vi "Version_2.0_Single_Column_Code.vi"() -> ()   [LabVIEW 2020] (continued)
                                n6800 = local read "VISA Refnum in\nfor Pump"() -> (w7287:refnum<visa-resource-name>)
                                n6801 = local write "Valve V5 Open"(FALSE ("Valve V1 Open")) -> ()
                                n6802 = local write "Suction pressure \nfor grid deposition"(w7284) -> ()
                                n6803 = local write "Re-deposit Sample\nonto Grid"(FALSE ("Redeposit Sample\nonto Grid")) -> ()
                                n6804 = local write "Pause Data Collection"(TRUE ("Pause Data Collection")) -> ()
                                n6805 = call "HardStopCurrentProcess (SubVI).vi"("VISA Refnum in"=w7287) -> ()  [unwired: 11 in]
                                n6806 = local write "Valve V6 Open"(TRUE ("Valve V2 Open")) -> ()
                                n6807 = local write "Valve V7 Open"(TRUE ("Valve V3 Open")) -> ()
                                }
                                frame #1 {
                                n6808 = call <vilib>:"fgt init.vi"() -> ("error out"=w7288:errorcluster)  [unwired: 11 in]
                                n6809 = while {
                                tunnel: [w7291] -> w7289
                                tunnel: w7288 -> [w7290]
                                stop <- w7294 stop-if-true
                                # "'5' corresponds to 2nd positin in the line-up series"
                                n6810 = local read "Stop for End of \nExperiment \nand Data Writing"() -> (w7295:bool)
                                n6811 = local read "Suction Pressure\nfor EM-grid \nDeposition (mbar)"() -> (w7292:sgl)
                                n6812 = call <vilib>:"fgt set pressure.vi"("error in (no error)"=w7290, "pressure"=w7292, "pressureIndex"=u32 1) -> ("error out"=w7291:errorcluster)  [unwired: 8 in]
                                n6813 = local read "Suction On/Off"() -> (w7297:bool)
                                n6814 = Not(x=w7297) -> (.not. x?=w7296:bool)
                                n6815 = Wait (ms)(milliseconds to wait=u32 10) -> ()  [unwired: 1 out]
                                n6816 = Or(x=w7296, y=w7295) -> (x .or. y?=w7294:bool)
                                }
                                n6817 = call <vilib>:"fgt close.vi"("error in (no error)"=w7289) -> ()  [unwired: 10 in, 1 out]
                                }
                                frame #2 {
                                n6818 = call <vilib>:"fgt init.vi"() -> ("error out"=w7300:errorcluster)  [unwired: 11 in]
                                n6819 = while {
                                tunnel: w7300 -> [w7303]
                                tunnel: [w7301] -> w7299
                                stop <- w7309 stop-if-true
                                n6820 = local read "Stop for End of \nExperiment \nand Data Writing"() -> (w7305:bool)
                                n6821 = local read "Suction On/Off"() -> (w7307:bool)
                                n6822 = call <vilib>:"fgt set pressure.vi"("error in (no error)"=w7303, "pressure"=sgl 0.0, "pressureIndex"=u32 1) -> ("error out"=w7301:errorcluster)  [unwired: 8 in]
                                n6823 = Not(x=w7307) -> (.not. x?=w7306:bool)
                                n6824 = Wait (ms)(milliseconds to wait=u32 10) -> ()  [unwired: 1 out]
                                n6825 = Or(x=w7306, y=w7305) -> (x .or. y?=w7309:bool)
                                }
                                n6826 = call <vilib>:"fgt close.vi"("error in (no error)"=w7299) -> ()  [unwired: 10 in, 1 out]
                                }
                                frame #3 {
                                n6827 = local write "Valve V7 Open"(FALSE ("Valve V3 Open")) -> ()
                                n6828 = local write "Valve V5 Open"(FALSE ("Valve V1 Open")) -> ()
                                n6829 = local write "Valve V6 Open"(FALSE ("Valve V2 Open")) -> ()
                                n6830 = local write "Valve V4 Open"(FALSE ("Valve V4 Open")) -> ()
                                }
                                frame #4 {
                                n6831 = while {
                                stop <- w7318 stop-if-true
                                n6832 = local read "Stop for End of \nExperiment \nand Data Writing"() -> (w7316:bool)
                                n6833 = local read "Re-deposit Sample\nonto Grid"() -> (w7319:bool)
                                n6834 = local read "Re-SEC"() -> (w7317:bool)
                                n6835 = Or(x=w7316, y=w7317) -> (x .or. y?=w7315:bool)
                                n6836 = Or(x=w7319, y=w7315) -> (x .or. y?=w7318:bool)
                                }
                                n6837 = One Button Dialog(message="Do you want to deposit sample on another grid? If yes, turn on 'Re-deposit Sample onto Grid'. Else turn on Re-SEC to do SEC again or STOP to end the experiment") -> ()  [unwired: 1 in, 1 out]
                                }
                                frame #5 {
                                n6838 = local write "Valve V4 Open"(TRUE ("Valve V4 Open")) -> ()
                                n6839 = local write "Valve V7 Open"(FALSE ("Valve V3 Open")) -> ()
                                n6840 = local write "Valve V5 Open"(TRUE ("Valve V1 Open")) -> ()
                                n6841 = local write "Valve V6 Open"(TRUE ("Valve V2 Open")) -> ()
                                }
                                frame #6 {
                                n6842 = local read "Re-deposit Sample\nonto Grid"() -> (w7324:bool)
                                n6843 = case shown="True" w7324 {
                                frame False {
                                n6844 = local write "Suction On/Off"(FALSE ("Suction On/Off")) -> ()
                                }
                                frame True {
                                n6845 = stacked-sequence {
                                frame #0 {
                                n6846 = local read "VISA Refnum in\nfor Pump"() -> (w7327:refnum<visa-resource-name>)
                                n6847 = call "AbsolutePlungerPosition (SubVI).vi"("VISA Refnum in"=w7327) -> ("Plunger Position"=w7326:i32)  [unwired: 10 in]
                                n6848 = local write "Position\nNow"(w7326) -> ()
                                }
                                frame #1 {
                                n6849 = local read "Buffer-C2 Pumping\nResolution"() -> (w7329:T2)
                                n6850 = case shown="\"Standard Pumping\", Default" w7329 {
                                tunnel: [w7330 w7341] -> w7328
                                frame "Standard Pumping", Default {
                                n6851 = local read "Buffer-C2 Volume \nto be Pumped"() -> (w7333:dbl)
                                n6852 = local read "Volume of Syringe"() -> (w7336:dbl)
                                n6853 = local read "Initial Plunger Position"() -> (w7340:dbl)
                                n6854 = local read "Position\nNow"() -> (w7339:dbl)
                                n6855 = Subtract(x=w7340, y=w7339) -> (x-y=w7338:dbl)
                                n6856 = Absolute Value(x=w7338) -> (abs(x)=w7337:dbl)
                                n6857 = Multiply(x=w7337, y=w7336) -> (x*y=w7335:dbl)
                                n6858 = Divide(x=w7335, y=3000.0) -> (x/y=w7332:dbl)
                                n6859 = Subtract(x=w7332, y=w7333) -> (x-y=w7331:dbl)
                                n6860 = Absolute Value(x=w7331) -> (abs(x)=w7330:dbl)
                                }
                                frame "High Resolution Pumping" {
                                n6861 = local read "Buffer-C2 Volume \nto be Pumped"() -> (w7344:dbl)
                                n6862 = local read "Volume of Syringe"() -> (w7347:dbl)
                                n6863 = local read "Initial Plunger Position"() -> (w7351:dbl)
                                n6864 = local read "Position\nNow"() -> (w7350:dbl)
                                n6865 = Subtract(x=w7351, y=w7350) -> (x-y=w7349:dbl)
                                n6866 = Absolute Value(x=w7349) -> (abs(x)=w7348:dbl)
                                n6867 = Multiply(x=w7348, y=w7347) -> (x*y=w7346:dbl)
                                n6868 = Divide(x=w7346, y=24000.0) -> (x/y=w7343:dbl)
                                n6869 = Subtract(x=w7343, y=w7344) -> (x-y=w7342:dbl)
                                n6870 = Absolute Value(x=w7342) -> (abs(x)=w7341:dbl)
                                }
                                }
                                n6871 = local write "Buffer-C Volume\nleft to be Pumped"(w7328) -> ()
                                }
                                frame #2 {
                                n6872 = local read "Buffer-C2 Dispense\nFlow Rate (ul/min)"() -> (w7355:dbl)
                                n6873 = local read "Buffer-C2 Pumping\nResolution"() -> (w7354:T2)
                                n6874 = local read "VISA Refnum in\nfor Pump"() -> (w7357:refnum<visa-resource-name>)
                                n6875 = local read "Volume of Syringe"() -> (w7356:dbl)
                                n6876 = call "GoToAbsolutePosition(SubVI).vi"("Absolute Volume Position in Syringe (in ul)"=0.0, "Volume of Syringe"=w7356, "Resolution of Pumping"=w7354, "Flow Rate (ul/min)"=w7355, "VISA Refnum in"=w7357) -> ()  [unwired: 6 in, 1 out]
                                n6877 = local write "Suction On/Off"(FALSE ("Suction On/Off")) -> ()
                                }
                                }
                                }
                                }
                                }
                                frame #7 {
                                n6878 = local read "Stop for End of \nExperiment \nand Data Writing"() -> (w7360:bool)
                                n6879 = local read "Re-SEC"() -> (w7359:bool)
                                n6880 = Or(x=w7360, y=w7359) -> (x .or. y?=w7358:bool)
                                n6881 = case shown="True" w7358 {
                                frame False {
                                }
                                frame True {
                                n6882 = local read "VISA Refnum in\nfor Pump"() -> (w7361:refnum<visa-resource-name>)
                                n6883 = call "HardStopCurrentProcess (SubVI).vi"("VISA Refnum in"=w7361) -> ()  [unwired: 11 in]
                                }
                                }
                                }
                                }
                                }
                                }
                                n6884 = local read "Stop for End of \nExperiment \nand Data Writing"() -> (w7207:bool)
                                n6885 = local read "Divert Sample \nonto Grid"() -> (w7210:bool)
                                n6886 = local read "Re-SEC"() -> (w7208:bool)
                                n6887 = Not(x=w7210) -> (.not. x?=w7209:bool)
                                n6888 = Or(x=w7207, y=w7208) -> (x .or. y?=w7206:bool)
                                n6889 = Or(x=w7209, y=w7206) -> (x .or. y?=w7211:bool)
                                }
                                }
                                }
                                n6890 = local write "Discard fluid \nprior to 1st \ndeposition"(TRUE ("Discard fluid \nprior to 1st \ndeposition")) -> ()
                                }
                                }
                                }
                                frame #34 {
                                n6891 = local read "VISA Refnum in\nfor Valve"() -> (w7363:refnum<visa-resource-name>)
                                n6892 = local read "External Valve \nOPEN"() -> (w7362:string)
                                n6893 = Wait (ms)(milliseconds to wait=u32 500) -> ()  [unwired: 1 out]
                                n6894 = call "PortChanger_Valve (SubVI).vi"("Port Number"=w7362, "VISA Refnum in"=w7363) -> ()  [unwired: 10 in]
                                }
                                frame #35 {
                                n6895 = local read "Stopper that ends \nthe main loops"() -> (w7366:bool)
                                n6896 = Wait (ms)(milliseconds to wait=u32 500) -> ()  [unwired: 1 out]
                                n6897 = case shown="True" w7366 {
                                frame False {
                                }
                                frame True {
                                n6898 = local read "VISA Refnum in\nfor Pump"() -> (w7370:refnum<visa-resource-name>)
                                n6899 = call "HardStopCurrentProcess (SubVI).vi"("VISA Refnum in"=w7370) -> ()  [unwired: 11 in]
                                }
                                }
                                n6900 = local write "Pause Data Collection"(TRUE ("Pause Data Collection")) -> ()
                                n6901 = local write "Start the Process"(FALSE ("Start the Process")) -> ()
                                n6902 = local write "Divert Sample \nonto Grid"(FALSE ("Divert Sample \nonto Grid")) -> ()
                                }
                                frame #36 {
                                n6903 = local read "Stop for End of \nExperiment \nand Data Writing"() -> (w7377:bool)
                                n6904 = local read "Start the Process"() -> (w7376:bool)
                                n6905 = Or(x=w7376, y=w7377) -> (x .or. y?=w7375:bool)
                                n6906 = case shown="True" w7375 {
                                frame False {
                                n6907 = while {
                                stop <- w7383 stop-if-true
                                n6908 = local read "Stop for End of \nExperiment \nand Data Writing"() -> (w7385:bool)
                                n6909 = local read "Start the Process"() -> (w7384:bool)
                                n6910 = Or(x=w7384, y=w7385) -> (x .or. y?=w7383:bool)
                                n6911 = Wait (ms)(milliseconds to wait=u32 100) -> ()  [unwired: 1 out]
                                }
                                n6912 = One Button Dialog(message="Do you want to re-introduce sample into column-2 and elute? If yes, adjust the re-introduction volume into column-2 and elution parameters for column-2 and turn on the 'Start the Process' button . If no, turn on the 'Stop for End of Experiment and Data Writing'.") -> ()  [unwired: 1 in, 1 out]
                                }
                                frame True {
                                n6913 = local read "Stop for End of \nExperiment \nand Data Writing"() -> (w7386:bool)
                                n6914 = case shown="True" w7386 {
                                frame False {
                                }
                                frame True {
                                n6915 = local write "Valve V1 Open"(FALSE ("Valve V1 Open")) -> ()
                                n6916 = local write "Valve V2 Open"(FALSE ("Valve V2 Open")) -> ()
                                n6917 = local write "Valve V3 Open"(FALSE ("Valve V3 Open")) -> ()
                                n6918 = local write "Valve V4 Open"(FALSE ("Valve V4 Open")) -> ()
                                n6919 = local write "Valve V5 Open"(FALSE ("Valve V5 Open")) -> ()
                                n6920 = local write "Valve V6 Open"(FALSE ("Valve V6 Open")) -> ()
                                n6921 = local write "Valve V7 Open"(FALSE ("Valve V7 Open")) -> ()
                                }
                                }
                                }
                                }
                                n6922 = local write "Sample Volume Diverted\ninto Column-2"(0.0 ("Sample Volume Diverted\ninto Column-2")) -> ()
                                n6923 = local write "Buffer-C Volume\nleft to be Pumped"(0.0 ("Buffer-C Volume\nleft to be Pumped")) -> ()
                                n6924 = local write "Vol_previous"(0.0 ("Vol_previous")) -> ()
                                n6925 = local write "Vol_now"(0.0 ("Vol_now")) -> ()
                                n6926 = local write "Volume being Injected \nin this process"(0.0 ("Volume being Injected \nin this process")) -> ()
                                n6927 = local write "Elution of Column-2"(FALSE ("Elution of Column-2")) -> ()
                                n6928 = local write "SEC On"(FALSE ("SEC On")) -> ()
                                }
                              }
                            }
                          }
                          n6929 = local read "Stop for End of \nExperiment \nand Data Writing"() -> (w6526:bool)
                        }
                      }
                    }
                  }
                }
              }
              frame True {
                n6930 = local write "Pause Data Collection"(FALSE ("Pause Data Collection")) -> ()
              }
            }
          }
          frame "Single Column Automated Protein Purification and Plunging" {
            n6931 = local read "Stopper that ends \nthe main loops"() -> (w7395:bool)
            n6932 = case shown="False" w7395 {
              frame False {
                n6933 = local read "Start the Process"() -> (w7396:bool)
                n6934 = case shown="True" w7396 {
                  frame False {
                    n6935 = local read "Stopper that ends \nthe main loops"() -> (w7398:bool)
                    n6936 = local read "Start the Process"() -> (w7397:bool)
                    n6937 = Or(x=w7398, y=w7397) -> (x .or. y?=w7399:bool)
                    n6938 = case shown="False" w7399 {
                      frame False {
                        n6939 = while {
                          stop <- w7402 stop-if-true
                          n6940 = local read "Stop for End of \nExperiment \nand Data Writing"() -> (w7401:bool)
                          n6941 = local read "Stopper that ends \nthe main loops"() -> (w7404:bool)
                          n6942 = local read "Start the Process"() -> (w7403:bool)
                          n6943 = Wait (ms)(milliseconds to wait=u32 10) -> ()  [unwired: 1 out]
                          n6944 = Or(x=w7404, y=w7403) -> (x .or. y?=w7402:bool)
                          n6945 = local write "Stopper that ends \nthe main loops"(w7401) -> ()
                        }
                        n6946 = One Button Dialog(message="Please Select the Process and Press 'Start the Process' Button") -> ()  [unwired: 1 in, 1 out]
                      }
                      frame True {
                      }
                    }
                  }
                  frame True {
                    n6947 = stacked-sequence {
                      frame #0 {
                        # "Equilibrate Column-1 with Buffer-A obtained from port-4 and pumped via port-2 and Column-2 with Buffer-C obtained from port-4 and pumped onto chip via port-6 onto the chip ...with an initial and inbetween wash of tubings while changing the buffers"
                        n6948 = stacked-sequence {
                          frame #0 {
                            n6949 = local write "Equilibriating \nColumn-1"(TRUE ("Equilibriating \nColumn-1")) -> ()
                            n6950 = local write "External Valve \nOpen"(FALSE ("External Valve \nOpen")) -> ()
                            n6951 = local write "Valve V1 Open"(FALSE ("Valve V1 Open")) -> ()
                            n6952 = local write "Valve V2 Open"(FALSE ("Valve V2 Open")) -> ()
                            n6953 = call <vilib>:"fgt init.vi"() -> ("error out"=w7409:errorcluster)  [unwired: 11 in]
                            n6954 = while {
                              tunnel: w7409 -> [w7413]
                              tunnel: [w7412] -> w7408
                              stop <- w7416 stop-if-true
                              # "Keeping the valve closing pressure of push pull to zero"
                              n6955 = local read "Stop for End of \nExperiment \nand Data Writing"() -> (w7417:bool)
                              n6956 = local read "Equilibriating \nColumn-1"() -> (w7418:bool)
                              n6957 = call <vilib>:"fgt set pressure.vi"("error in (no error)"=w7413, "pressure"=sgl 0.0 ("order"), "pressureIndex"=1 ("module")) -> ("error out"=w7412:errorcluster)  [unwired: 8 in]
                              n6958 = Or(x=w7418, y=w7417) -> (x .or. y?=w7416:bool)
                              n6959 = Wait (ms)(milliseconds to wait=u32 10) -> ()  [unwired: 1 out]
                            }
                            n6960 = call <vilib>:"fgt close.vi"("error in (no error)"=w7408) -> ()  [unwired: 10 in, 1 out]
                          }
                          frame #1 {
                            # "Clean the elution tubing with Buffer-B1"
                            n6961 = local read "N-B1"() -> (w7420:i32)
                            n6962 = for {
                              N: w7420 -> [_]
                              n6963 = stacked-sequence {
                                frame #0 {
                                n6964 = local read "VISA Refnum in\nfor Pump"() -> (w7423:refnum<visa-resource-name>)
                                n6965 = local read "Port for \nB-Elution"() -> (w7422:string)
                                n6966 = call "PortChanger (SubVI).vi"("Port Number"=w7422, "VISA Refnum in"=w7423) -> ()  [unwired: 10 in]
                                }
                                frame #1 {
                                n6967 = local read "VISA Refnum in\nfor Pump"() -> (w7424:refnum<visa-resource-name>)
                                n6968 = call "ProcessCompletionWaiter (SubVI).vi"("VISA Refnum in"=w7424) -> ()  [unwired: 11 in]
                                }
                                frame #2 {
                                n6969 = local read "VISA Refnum in\nfor Pump"() -> (w7429:refnum<visa-resource-name>)
                                n6970 = local read "Apparent Volume\nof Syringe"() -> (w7425:dbl)
                                n6971 = local read "Volume of Syringe"() -> (w7426:dbl)
                                n6972 = call "RPickUp(SubVI).vi"("Volume to be picked up"=w7425, "Volume of Syringe"=w7426, "Resolution of PickUP"=T2."Standard Pumping", "PickUp Flow Rate (ul/min)"=150.0, "VISA Refnum in"=w7429) -> ()  [unwired: 6 in, 1 out]
                                }
                                frame #3 {
                                n6973 = local read "Stopper that ends \nthe main loops"() -> (w7430:bool)
                                n6974 = local read "VISA Refnum in\nfor Pump"() -> (w7431:refnum<visa-resource-name>)
                                n6975 = case shown="True" w7430 {
                                frame False {
                                }
                                frame True {
                                n6976 = local read "VISA Refnum in\nfor Pump"() -> (w7432:refnum<visa-resource-name>)
                                n6977 = call "HardStopCurrentProcess (SubVI).vi"("VISA Refnum in"=w7432) -> ()  [unwired: 11 in]
                                }
                                }
                                n6978 = call "ProcessCompletionWaiter (SubVI).vi"("VISA Refnum in"=w7431) -> ()  [unwired: 11 in]
                                }
                                frame #4 {
                                n6979 = local read "VISA Refnum in\nfor Pump"() -> (w7434:refnum<visa-resource-name>)
                                n6980 = call "PortChanger (SubVI).vi"("Port Number"="1", "VISA Refnum in"=w7434) -> ()  [unwired: 10 in]
                                }
                                frame #5 {
                                n6981 = local read "Stopper that ends \nthe main loops"() -> (w7435:bool)
                                n6982 = local read "VISA Refnum in\nfor Pump"() -> (w7436:refnum<visa-resource-name>)
                                n6983 = case shown="True" w7435 {
                                frame False {
                                }
                                frame True {
                                n6984 = local read "VISA Refnum in\nfor Pump"() -> (w7437:refnum<visa-resource-name>)
                                n6985 = call "HardStopCurrentProcess (SubVI).vi"("VISA Refnum in"=w7437) -> ()  [unwired: 11 in]
                                }
                                }
                                n6986 = call "ProcessCompletionWaiter (SubVI).vi"("VISA Refnum in"=w7436) -> ()  [unwired: 11 in]
                                }
                                frame #6 {
                                n6987 = local read "VISA Refnum in\nfor Pump"() -> (w7442:refnum<visa-resource-name>)
                                n6988 = local read "Volume of Syringe"() -> (w7439:dbl)
                                n6989 = call "GoToAbsolutePosition(SubVI).vi"("Absolute Volume Position in Syringe (in ul)"=0.0 ("Volume to be picked up"), "Volume of Syringe"=w7439, "Resolution of Pumping"=T2."Standard Pumping" ("Resolution of PickUP"), "Flow Rate (ul/min)"=150.0 ("PickUp Flow Rate (ul/min)"), "VISA Refnum in"=w7442) -> ()  [unwired: 6 in, 1 out]
                                }
                                frame #7 {
                                n6990 = local read "Stopper that ends \nthe main loops"() -> (w7443:bool)
                                n6991 = local read "VISA Refnum in\nfor Pump"() -> (w7444:refnum<visa-resource-name>)
                                n6992 = case shown="True" w7443 {
                                frame False {
                                }
                                frame True {
                                n6993 = local read "VISA Refnum in\nfor Pump"() -> (w7445:refnum<visa-resource-name>)
                                n6994 = call "HardStopCurrentProcess (SubVI).vi"("VISA Refnum in"=w7445) -> ()  [unwired: 11 in]
                                }
                                }
                                n6995 = call "ProcessCompletionWaiter (SubVI).vi"("VISA Refnum in"=w7444) -> ()  [unwired: 11 in]
                                }
                              }
                              n6996 = local write "Pause Data Collection"(TRUE ("Pause Data Collection")) -> ()
                            }
                          }
                          frame #2 {
                            # "Switch to Port-7"
                            # "Port-7 of pump is connected to Buffer-B"
                            n6997 = local read "VISA Refnum in\nfor Pump"() -> (w7447:refnum<visa-resource-name>)
                            n6998 = local read "Port for \nB-Elution"() -> (w7446:string)
                            n6999 = call "PortChanger (SubVI).vi"("Port Number"=w7446, "VISA Refnum in"=w7447) -> ()  [unwired: 10 in]
                          }
                          frame #3 {
                            n7000 = local read "VISA Refnum in\nfor Pump"() -> (w7448:refnum<visa-resource-name>)
                            n7001 = call "ProcessCompletionWaiter (SubVI).vi"("VISA Refnum in"=w7448) -> ()  [unwired: 11 in]
                          }
                          frame #4 {
                            # "External vale is temporarily connected to teh waste outlet in this code"
                            n7002 = local write "Valve V1 Open"(FALSE ("Valve V1 Open")) -> ()
                            n7003 = local write "Valve V2 Open"(TRUE ("Valve V2 Open")) -> ()
                            n7004 = local write "External Valve \nOpen"(TRUE ("External Valve \nOpen")) -> ()
                          }
                          frame #5 {
                            n7005 = local read "Apparent Volume\nof Syringe"() -> (w7452:dbl)
                            n7006 = local read "Buffer-B Volume \nfor elution tubing \npre-wash"() -> (w7455:dbl)
                            n7007 = Quotient & Remainder(x=w7455, y=w7452) -> (x-y*floor(x/y)=w7453:dbl, floor(x/y)=w7454:dbl)
                            n7008 = for {
                              N: w7454 -> [_]
                              n7009 = stacked-sequence {
                                frame #0 {
                                n7010 = local read "Buffer-B PickUp \nFlow Rate (ul/min)"() -> (w7458:dbl)
                                n7011 = local read "Buffer-B Pumping\nResolution"() -> (w7457:T2)
                                n7012 = local read "VISA Refnum in\nfor Pump"() -> (w7460:refnum<visa-resource-name>)
                                n7013 = local read "Apparent Volume\nof Syringe"() -> (w7456:dbl)
                                n7014 = local read "Volume of Syringe"() -> (w7459:dbl)
                                n7015 = call "RPickUp(SubVI).vi"("Volume to be picked up"=w7456, "Volume of Syringe"=w7459, "Resolution of PickUP"=w7457, "PickUp Flow Rate (ul/min)"=w7458, "VISA Refnum in"=w7460) -> ()  [unwired: 6 in, 1 out]
                                }
                                frame #1 {
                                n7016 = while {
                                stop <- w7461 stop-if-true
                                n7017 = local read "Stopper that ends \nthe main loops"() -> (w7462:bool)
                                n7018 = local read "VISA Refnum in\nfor Pump"() -> (w7463:refnum<visa-resource-name>)
                                n7019 = case shown="True" w7462 {
                                frame False {
                                }
                                frame True {
                                n7020 = local read "VISA Refnum in\nfor Pump"() -> (w7464:refnum<visa-resource-name>)
                                n7021 = call "HardStopCurrentProcess (SubVI).vi"("VISA Refnum in"=w7464) -> ()  [unwired: 11 in]
                                }
                                }
                                n7022 = call "ProcessCompletionWaiterWithOutPut (SubVI).vi"("VISA Refnum in"=w7463) -> ("Boolean"=w7461:bool)  [unwired: 10 in]
                                }
                                }
                                frame #2 {
                                # "Reads the initial Plunger Position for computing the volume dispensed"
                                n7023 = local read "VISA Refnum in\nfor Pump"() -> (w7466:refnum<visa-resource-name>)
                                n7024 = call "AbsolutePlungerPosition (SubVI).vi"("VISA Refnum in"=w7466) -> ("Plunger Position"=w7465:i32)  [unwired: 10 in]
                                n7025 = local write "Initial Plunger Position"(w7465) -> ()
                                }
                                frame #3 {
                                # "Switch to Port-8"
                                # "Port-8 of the pump is conncted to elution tubing for column-1 of chip"
                                n7026 = local read "VISA Refnum in\nfor Pump"() -> (w7468:refnum<visa-resource-name>)
                                n7027 = call "PortChanger (SubVI).vi"("Port Number"="8", "VISA Refnum in"=w7468) -> ()  [unwired: 10 in]
                                }
                                frame #4 {
                                n7028 = while {
                                stop <- w7469 stop-if-true
                                n7029 = local read "Stopper that ends \nthe main loops"() -> (w7470:bool)
                                n7030 = local read "VISA Refnum in\nfor Pump"() -> (w7471:refnum<visa-resource-name>)
                                n7031 = case shown="True" w7470 {
                                frame False {
                                }
                                frame True {
                                n7032 = local read "VISA Refnum in\nfor Pump"() -> (w7472:refnum<visa-resource-name>)
                                n7033 = call "HardStopCurrentProcess (SubVI).vi"("VISA Refnum in"=w7472) -> ()  [unwired: 11 in]
                                }
                                }
                                n7034 = call "ProcessCompletionWaiterWithOutPut (SubVI).vi"("VISA Refnum in"=w7471) -> ("Boolean"=w7469:bool)  [unwired: 10 in]
                                }
                                }
                                frame #5 {
                                n7035 = local read "Buffer-B Dispense\nFlow Rate for Elution \ntubing pre-wash"() -> (w7476:dbl)
                                n7036 = local read "Buffer-B Pumping\nResolution"() -> (w7475:T2)
                                n7037 = local read "VISA Refnum in\nfor Pump"() -> (w7478:refnum<visa-resource-name>)
                                n7038 = local write "Pause Data Collection"(TRUE ("Pause Data Collection")) -> ()
                                n7039 = local read "Volume of Syringe"() -> (w7477:dbl)
                                n7040 = call "GoToAbsolutePosition(SubVI).vi"("Absolute Volume Position in Syringe (in ul)"=0.0, "Volume of Syringe"=w7477, "Resolution of Pumping"=w7475, "Flow Rate (ul/min)"=w7476, "VISA Refnum in"=w7478) -> ()  [unwired: 6 in, 1 out]
                                }
                                frame #6 {
                                n7041 = local read "VISA Refnum in\nfor Pump"() -> (w7482:refnum<visa-resource-name>)
                                n7042 = local read "Initial Plunger Position"() -> (w7481:dbl)
                                n7043 = local read "Volume of Syringe"() -> (w7479:dbl)
                                n7044 = local read "Buffer-B Pumping\nResolution"() -> (w7480:T2)
                                n7045 = while {
                                tunnel: w7481 -> [w7489]
                                tunnel: w7482 -> [w7488]
                                tunnel: w7480 -> [w7487]
                                tunnel: w7479 -> [w7486]
                                stop <- w7484 stop-if-true
                                n7046 = stacked-sequence {
                                tunnel: w7489 -> [w7496 _]
                                tunnel: w7488 -> [w7495 w7516]
                                tunnel: w7487 -> [w7494 _]
                                tunnel: w7486 -> [w7493 _]
                                tunnel: [_ w7514] -> w7484
                                frame #0 {
                                n7047 = call "AbsolutePlungerPosition (SubVI).vi"("VISA Refnum in"=w7495) -> ("Plunger Position"=w7492:i32)  [unwired: 10 in]
                                n7048 = case shown="\"Standard Pumping\", Default" w7494 {
                                tunnel: w7496 -> [w7501 w7510]
                                tunnel: w7492 -> [w7502 w7509]
                                tunnel: [w7500 w7507] -> w7491
                                tunnel: w7493 -> [w7499 w7508]
                                frame "Standard Pumping", Default {
                                n7049 = Subtract(x=w7501, y=w7502) -> (x-y=w7498:dbl)
                                n7050 = Absolute Value(x=w7498) -> (abs(x)=w7497:dbl)
                                n7051 = Multiply(x=w7497, y=w7499) -> (x*y=w7504:dbl)
                                n7052 = Divide(x=w7504, y=3000.0) -> (x/y=w7500:dbl)
                                }
                                frame "High Resolution Pumping" {
                                n7053 = Subtract(x=w7510, y=w7509) -> (x-y=w7506:dbl)
                                n7054 = Absolute Value(x=w7506) -> (abs(x)=w7505:dbl)
                                n7055 = Multiply(x=w7505, y=w7508) -> (x*y=w7512:dbl)
                                n7056 = Divide(x=w7512, y=24000.0) -> (x/y=w7507:dbl)
                                }
                                }
                                n7057 = local write "Volume being Injected \nin this process"(w7491) -> ()
                                }
                                frame #1 {
                                n7058 = call "LSPOneStatus (SubVI).vi"("VISA Refnum in"=w7516) -> ("read buffer"=w7518:string)  [unwired: 10 in]
                                n7059 = call <vilib>:"Trim Whitespace.vi"("string"=w7518) -> ("trimmed string"=w7517:string)  [unwired: 1 in]
                                n7060 = local read "Stopper that ends \nthe main loops"() -> (w7513:bool)
                                n7061 = Equal?(x=w7517, y="/0`\u0003") -> (x = y?=w7515:bool)
                                n7062 = Or(x=w7515, y=w7513) -> (x .or. y?=w7514:bool)
                                }
                                }
                                n7063 = Wait (ms)(milliseconds to wait=u32 100) -> ()  [unwired: 1 out]
                                n7064 = local read "Stopper that ends \nthe main loops"() -> (w7483:bool)
                                n7065 = case shown="True" w7483 {
                                frame False {
                                }
                                frame True {
                                n7066 = local read "VISA Refnum in\nfor Pump"() -> (w7490:refnum<visa-resource-name>)
                                n7067 = call "HardStopCurrentProcess (SubVI).vi"("VISA Refnum in"=w7490) -> ()  [unwired: 11 in]
                                }
                                }
                                }
                                }
                                frame #7 {
                                # "Change the pump port back to Buffer-B"
                                n7068 = local read "VISA Refnum in\nfor Pump"() -> (w7521:refnum<visa-resource-name>)
                                n7069 = local read "Port for \nB-Elution"() -> (w7520:string)
                                n7070 = local write "Pause Data Collection"(TRUE ("Pause Data Collection")) -> ()
                                n7071 = Wait (ms)(milliseconds to wait=u32 500) -> ()  [unwired: 1 out]
                                n7072 = call "PortChanger (SubVI).vi"("Port Number"=w7520, "VISA Refnum in"=w7521) -> ()  [unwired: 10 in]
                                }
                                frame #8 {
                                n7073 = local read "VISA Refnum in\nfor Pump"() -> (w7524:refnum<visa-resource-name>)
                                n7074 = local write "Volume being Injected \nin this process"(0.0 ("Volume being Injected \nin this process")) -> ()
                                n7075 = call "ProcessCompletionWaiter (SubVI).vi"("VISA Refnum in"=w7524) -> ()  [unwired: 11 in]
                                }
                              }
                            }
                            n7076 = local write "Reminder of the \nVolume to be \nPumped"(w7453) -> ()
                          }
                          frame #6 {
                            n7077 = stacked-sequence {
                              frame #0 {
                                n7078 = local read "Buffer-B PickUp \nFlow Rate (ul/min)"() -> (w7528:dbl)
                                n7079 = local read "Buffer-B Pumping\nResolution"() -> (w7527:T2)
                                n7080 = local read "VISA Refnum in\nfor Pump"() -> (w7530:refnum<visa-resource-name>)
                                n7081 = local read "Reminder of the \nVolume to be \nPumped"() -> (w7526:dbl)
                                n7082 = local read "Volume of Syringe"() -> (w7529:dbl)
                                n7083 = call "RPickUp(SubVI).vi"("Volume to be picked up"=w7526, "Volume of Syringe"=w7529, "Resolution of PickUP"=w7527, "PickUp Flow Rate (ul/min)"=w7528, "VISA Refnum in"=w7530) -> ()  [unwired: 6 in, 1 out]
                              }
                              frame #1 {
                                n7084 = while {
                                stop <- w7531 stop-if-true
                                n7085 = local read "Stopper that ends \nthe main loops"() -> (w7532:bool)
                                n7086 = local read "VISA Refnum in\nfor Pump"() -> (w7533:refnum<visa-resource-name>)
                                n7087 = case shown="True" w7532 {
                                frame False {
                                }
                                frame True {
                                n7088 = local read "VISA Refnum in\nfor Pump"() -> (w7534:refnum<visa-resource-name>)
                                n7089 = call "HardStopCurrentProcess (SubVI).vi"("VISA Refnum in"=w7534) -> ()  [unwired: 11 in]
                                }
                                }
                                n7090 = call "ProcessCompletionWaiterWithOutPut (SubVI).vi"("VISA Refnum in"=w7533) -> ("Boolean"=w7531:bool)  [unwired: 10 in]
                                }
                              }
                              frame #2 {
                                # "Reads the initial Plunger Position for computing the volume dispensed"
                                n7091 = local read "VISA Refnum in\nfor Pump"() -> (w7536:refnum<visa-resource-name>)
                                n7092 = call "AbsolutePlungerPosition (SubVI).vi"("VISA Refnum in"=w7536) -> ("Plunger Position"=w7535:i32)  [unwired: 10 in]
                                n7093 = local write "Initial Plunger Position"(w7535) -> ()
                              }
                              frame #3 {
                                # "Switch to Port-8"
                                # "Port-8 of the pump is conncted to elution inlet of column-1 of chip"
                                n7094 = local read "VISA Refnum in\nfor Pump"() -> (w7538:refnum<visa-resource-name>)
                                n7095 = call "PortChanger (SubVI).vi"("Port Number"="8", "VISA Refnum in"=w7538) -> ()  [unwired: 10 in]
                              }
                              frame #4 {
                                n7096 = while {
                                stop <- w7539 stop-if-true
                                n7097 = local read "Stopper that ends \nthe main loops"() -> (w7540:bool)
                                n7098 = local read "VISA Refnum in\nfor Pump"() -> (w7541:refnum<visa-resource-name>)
                                n7099 = case shown="True" w7540 {
                                frame False {
                                }
                                frame True {
                                n7100 = local read "VISA Refnum in\nfor Pump"() -> (w7542:refnum<visa-resource-name>)
                                n7101 = call "HardStopCurrentProcess (SubVI).vi"("VISA Refnum in"=w7542) -> ()  [unwired: 11 in]
                                }
                                }
                                n7102 = call "ProcessCompletionWaiterWithOutPut (SubVI).vi"("VISA Refnum in"=w7541) -> ("Boolean"=w7539:bool)  [unwired: 10 in]
                                }
                              }
                              frame #5 {
                                n7103 = local read "Buffer-B Dispense\nFlow Rate for Elution \ntubing pre-wash"() -> (w7546:dbl)
                                n7104 = local read "Buffer-B Pumping\nResolution"() -> (w7545:T2)
                                n7105 = local read "VISA Refnum in\nfor Pump"() -> (w7548:refnum<visa-resource-name>)
                                n7106 = local write "Pause Data Collection"(TRUE ("Pause Data Collection")) -> ()
                                n7107 = local read "Volume of Syringe"() -> (w7547:dbl)
                                n7108 = call "GoToAbsolutePosition(SubVI).vi"("Absolute Volume Position in Syringe (in ul)"=0.0 ("Volume to be Dispensed"), "Volume of Syringe"=w7547, "Resolution of Pumping"=w7545, "Flow Rate (ul/min)"=w7546, "VISA Refnum in"=w7548) -> ()  [unwired: 6 in, 1 out]
                              }
                              frame #6 {
                                n7109 = local read "VISA Refnum in\nfor Pump"() -> (w7552:refnum<visa-resource-name>)
                                n7110 = local read "Initial Plunger Position"() -> (w7551:dbl)
                                n7111 = local read "Volume of Syringe"() -> (w7549:dbl)
                                n7112 = local read "Buffer-B Pumping\nResolution"() -> (w7550:T2)
                                n7113 = while {
                                tunnel: w7551 -> [w7559]
                                tunnel: w7552 -> [w7558]
                                tunnel: w7550 -> [w7557]
                                tunnel: w7549 -> [w7556]
                                stop <- w7554 stop-if-true
                                n7114 = stacked-sequence {
                                tunnel: w7559 -> [w7566 _]
                                tunnel: w7558 -> [w7565 w7586]
                                tunnel: w7557 -> [w7564 _]
                                tunnel: w7556 -> [w7563 _]
                                tunnel: [_ w7584] -> w7554
                                frame #0 {
                                n7115 = call "AbsolutePlungerPosition (SubVI).vi"("VISA Refnum in"=w7565) -> ("Plunger Position"=w7562:i32)  [unwired: 10 in]
                                n7116 = case shown="\"Standard Pumping\", Default" w7564 {
                                tunnel: w7566 -> [w7571 w7580]
                                tunnel: w7562 -> [w7572 w7579]
                                tunnel: [w7570 w7577] -> w7561
                                tunnel: w7563 -> [w7569 w7578]
                                frame "Standard Pumping", Default {
                                n7117 = Subtract(x=w7571, y=w7572) -> (x-y=w7568:dbl)
                                n7118 = Absolute Value(x=w7568) -> (abs(x)=w7567:dbl)
                                n7119 = Multiply(x=w7567, y=w7569) -> (x*y=w7574:dbl)
                                n7120 = Divide(x=w7574, y=3000.0) -> (x/y=w7570:dbl)
                                }
                                frame "High Resolution Pumping" {
                                n7121 = Subtract(x=w7580, y=w7579) -> (x-y=w7576:dbl)
                                n7122 = Absolute Value(x=w7576) -> (abs(x)=w7575:dbl)
                                n7123 = Multiply(x=w7575, y=w7578) -> (x*y=w7582:dbl)
                                n7124 = Divide(x=w7582, y=24000.0) -> (x/y=w7577:dbl)
                                }
                                }
                                n7125 = local write "Volume being Injected \nin this process"(w7561) -> ()
                                }
                                frame #1 {
                                n7126 = call "LSPOneStatus (SubVI).vi"("VISA Refnum in"=w7586) -> ("read buffer"=w7588:string)  [unwired: 10 in]
                                n7127 = call <vilib>:"Trim Whitespace.vi"("string"=w7588) -> ("trimmed string"=w7587:string)  [unwired: 1 in]
                                n7128 = local read "Stopper that ends \nthe main loops"() -> (w7583:bool)
                                n7129 = Equal?(x=w7587, y="/0`\u0003") -> (x = y?=w7585:bool)
                                n7130 = Or(x=w7585, y=w7583) -> (x .or. y?=w7584:bool)
                                }
                                }
                                n7131 = Wait (ms)(milliseconds to wait=u32 100) -> ()  [unwired: 1 out]
                                n7132 = local read "Stopper that ends \nthe main loops"() -> (w7553:bool)
                                n7133 = case shown="True" w7553 {
                                frame False {
                                }
                                frame True {
                                n7134 = local read "VISA Refnum in\nfor Pump"() -> (w7560:refnum<visa-resource-name>)
                                n7135 = call "HardStopCurrentProcess (SubVI).vi"("VISA Refnum in"=w7560) -> ()  [unwired: 11 in]
                                }
                                }
                                }
                              }
                              frame #7 {
                                # "Change the pump port to Buffer-A1 for equilibriation of column-1"
                                n7136 = local read "VISA Refnum in\nfor Pump"() -> (w7591:refnum<visa-resource-name>)
                                n7137 = local read "Port for \nA1-Equilibriation"() -> (w7590:string)
                                n7138 = local write "Pause Data Collection"(TRUE ("Pause Data Collection")) -> ()
                                n7139 = Wait (ms)(milliseconds to wait=u32 500) -> ()  [unwired: 1 out]
                                n7140 = call "PortChanger (SubVI).vi"("Port Number"=w7590, "VISA Refnum in"=w7591) -> ()  [unwired: 10 in]
                              }
                              frame #8 {
                                n7141 = local read "VISA Refnum in\nfor Pump"() -> (w7595:refnum<visa-resource-name>)
                                n7142 = local write "Volume being Injected \nin this process"(0.0 ("Volume being Injected \nin this process")) -> ()
                                n7143 = call "ProcessCompletionWaiter (SubVI).vi"("VISA Refnum in"=w7595) -> ()  [unwired: 11 in]
                                n7144 = local write "Start the Process"(FALSE ("Start the Process")) -> ()
                              }
                            }
                          }
                          frame #7 {
                            # "Clean the tubing with Buffer-A1"
                            n7145 = local read "N-A1"() -> (w7597:i32)
                            n7146 = for {
                              N: w7597 -> [_]
                              n7147 = stacked-sequence {
                                frame #0 {
                                n7148 = local read "VISA Refnum in\nfor Pump"() -> (w7600:refnum<visa-resource-name>)
                                n7149 = local read "Port for \nA1-Equilibriation"() -> (w7599:string)
                                n7150 = call "PortChanger (SubVI).vi"("Port Number"=w7599, "VISA Refnum in"=w7600) -> ()  [unwired: 10 in]
                                }
                                frame #1 {
                                n7151 = local read "VISA Refnum in\nfor Pump"() -> (w7601:refnum<visa-resource-name>)
                                n7152 = call "ProcessCompletionWaiter (SubVI).vi"("VISA Refnum in"=w7601) -> ()  [unwired: 11 in]
                                }
                                frame #2 {
                                n7153 = local read "VISA Refnum in\nfor Pump"() -> (w7606:refnum<visa-resource-name>)
                                n7154 = local read "Apparent Volume\nof Syringe"() -> (w7602:dbl)
                                n7155 = local read "Volume of Syringe"() -> (w7603:dbl)
                                n7156 = call "RPickUp(SubVI).vi"("Volume to be picked up"=w7602, "Volume of Syringe"=w7603, "Resolution of PickUP"=T2."Standard Pumping", "PickUp Flow Rate (ul/min)"=150.0, "VISA Refnum in"=w7606) -> ()  [unwired: 6 in, 1 out]
                                }
                                frame #3 {
                                n7157 = local read "Stopper that ends \nthe main loops"() -> (w7607:bool)
                                n7158 = local read "VISA Refnum in\nfor Pump"() -> (w7608:refnum<visa-resource-name>)
                                n7159 = case shown="True" w7607 {
                                frame False {
                                }
                                frame True {
                                n7160 = local read "VISA Refnum in\nfor Pump"() -> (w7609:refnum<visa-resource-name>)
                                n7161 = call "HardStopCurrentProcess (SubVI).vi"("VISA Refnum in"=w7609) -> ()  [unwired: 11 in]
                                }
                                }
                                n7162 = call "ProcessCompletionWaiter (SubVI).vi"("VISA Refnum in"=w7608) -> ()  [unwired: 11 in]
                                }
                                frame #4 {
                                n7163 = local read "VISA Refnum in\nfor Pump"() -> (w7611:refnum<visa-resource-name>)
                                n7164 = call "PortChanger (SubVI).vi"("Port Number"="1", "VISA Refnum in"=w7611) -> ()  [unwired: 10 in]
                                }
                                frame #5 {
                                n7165 = local read "Stopper that ends \nthe main loops"() -> (w7612:bool)
                                n7166 = local read "VISA Refnum in\nfor Pump"() -> (w7613:refnum<visa-resource-name>)
                                n7167 = case shown="True" w7612 {
                                frame False {
                                }
                                frame True {
                                n7168 = local read "VISA Refnum in\nfor Pump"() -> (w7614:refnum<visa-resource-name>)
                                n7169 = call "HardStopCurrentProcess (SubVI).vi"("VISA Refnum in"=w7614) -> ()  [unwired: 11 in]
                                }
                                }
                                n7170 = call "ProcessCompletionWaiter (SubVI).vi"("VISA Refnum in"=w7613) -> ()  [unwired: 11 in]
                                }
                                frame #6 {
                                n7171 = local read "VISA Refnum in\nfor Pump"() -> (w7619:refnum<visa-resource-name>)
                                n7172 = local read "Volume of Syringe"() -> (w7616:dbl)
                                n7173 = call "GoToAbsolutePosition(SubVI).vi"("Absolute Volume Position in Syringe (in ul)"=0.0 ("Volume to be picked up"), "Volume of Syringe"=w7616, "Resolution of Pumping"=T2."Standard Pumping" ("Resolution of PickUP"), "Flow Rate (ul/min)"=150.0 ("PickUp Flow Rate (ul/min)"), "VISA Refnum in"=w7619) -> ()  [unwired: 6 in, 1 out]
                                }
                                frame #7 {
                                n7174 = local read "Stopper that ends \nthe main loops"() -> (w7620:bool)
                                n7175 = local read "VISA Refnum in\nfor Pump"() -> (w7621:refnum<visa-resource-name>)
                                n7176 = case shown="True" w7620 {
                                frame False {
                                }
                                frame True {
                                n7177 = local read "VISA Refnum in\nfor Pump"() -> (w7622:refnum<visa-resource-name>)
                                n7178 = call "HardStopCurrentProcess (SubVI).vi"("VISA Refnum in"=w7622) -> ()  [unwired: 11 in]
                                }
                                }
                                n7179 = call "ProcessCompletionWaiter (SubVI).vi"("VISA Refnum in"=w7621) -> ()  [unwired: 11 in]
                                }
                              }
                              n7180 = local write "Pause Data Collection"(TRUE ("Pause Data Collection")) -> ()
                            }
                          }
                          frame #8 {
                            # "Switch to Port-4"
                            # "Port-4 of pump is connected to Buffer-A1"
                            n7181 = local read "Port for \nA1-Equilibriation"() -> (w7623:string)
                            n7182 = local read "VISA Refnum in\nfor Pump"() -> (w7624:refnum<visa-resource-name>)
                            n7183 = call "PortChanger (SubVI).vi"("Port Number"=w7623, "VISA Refnum in"=w7624) -> ()  [unwired: 10 in]
                          }
                          frame #9 {
                            n7184 = local read "VISA Refnum in\nfor Pump"() -> (w7625:refnum<visa-resource-name>)
                            n7185 = call "ProcessCompletionWaiter (SubVI).vi"("VISA Refnum in"=w7625) -> ()  [unwired: 11 in]
                          }
                          frame #10 {
                            # "External vale is temporarily connected to teh waste outlet in this code"
                            n7186 = local write "Valve V1 Open"(TRUE ("Valve V1 Open")) -> ()
                            n7187 = local write "Valve V2 Open"(FALSE ("Valve V2 Open")) -> ()
                            n7188 = local write "External Valve \nOpen"(FALSE ("External Valve \nOpen")) -> ()
                          }
                          frame #11 {
                            n7189 = local read "Buffer-A1 Volume \nto be  Pumped \nfor Equilibration\nof Column-1"() -> (w7632:dbl)
                            n7190 = local read "Apparent Volume\nof Syringe"() -> (w7629:dbl)
                            n7191 = Quotient & Remainder(x=w7632, y=w7629) -> (x-y*floor(x/y)=w7630:dbl, floor(x/y)=w7631:dbl)
                            n7192 = for {
                              N: w7631 -> [_]
                              n7193 = stacked-sequence {
                                frame #0 {
                                n7194 = local read "Buffer-A1 PickUp \nFlow Rate (ul/min)\nfor Equilibration \nof Column-1"() -> (w7635:dbl)
                                n7195 = local read "Buffer-A1 Pumping\nResolution \nfor Equilibration \nof Column-1"() -> (w7634:T2)
                                n7196 = local read "VISA Refnum in\nfor Pump"() -> (w7637:refnum<visa-resource-name>)
                                n7197 = local read "Apparent Volume\nof Syringe"() -> (w7633:dbl)
                                n7198 = local read "Volume of Syringe"() -> (w7636:dbl)
                                n7199 = call "RPickUp(SubVI).vi"("Volume to be picked up"=w7633, "Volume of Syringe"=w7636, "Resolution of PickUP"=w7634, "PickUp Flow Rate (ul/min)"=w7635, "VISA Refnum in"=w7637) -> ()  [unwired: 6 in, 1 out]
                                }
                                frame #1 {
                                n7200 = while {
                                stop <- w7638 stop-if-true
                                n7201 = local read "Stopper that ends \nthe main loops"() -> (w7639:bool)
                                n7202 = local read "VISA Refnum in\nfor Pump"() -> (w7640:refnum<visa-resource-name>)
                                n7203 = case shown="True" w7639 {
                                frame False {
                                }
                                frame True {
                                n7204 = local read "VISA Refnum in\nfor Pump"() -> (w7641:refnum<visa-resource-name>)
                                n7205 = call "HardStopCurrentProcess (SubVI).vi"("VISA Refnum in"=w7641) -> ()  [unwired: 11 in]
                                }
                                }
                                n7206 = call "ProcessCompletionWaiterWithOutPut (SubVI).vi"("VISA Refnum in"=w7640) -> ("Boolean"=w7638:bool)  [unwired: 10 in]
                                }
                                }
                                frame #2 {
                                # "Reads the initial Plunger Position for computing the volume dispensed"
                                n7207 = local read "VISA Refnum in\nfor Pump"() -> (w7643:refnum<visa-resource-name>)
                                n7208 = call "AbsolutePlungerPosition (SubVI).vi"("VISA Refnum in"=w7643) -> ("Plunger Position"=w7642:i32)  [unwired: 10 in]
                                n7209 = local write "Initial Plunger Position"(w7642) -> ()
                                }
                                frame #3 {
                                # "Switch to Port-2"
                                # "Port-2 of the pump is conncted to column-1 of chip"
                                n7210 = local read "VISA Refnum in\nfor Pump"() -> (w7645:refnum<visa-resource-name>)
                                n7211 = call "PortChanger (SubVI).vi"("Port Number"="2", "VISA Refnum in"=w7645) -> ()  [unwired: 10 in]
                                }
                                frame #4 {
                                n7212 = while {
                                stop <- w7646 stop-if-true
                                n7213 = local read "Stopper that ends \nthe main loops"() -> (w7647:bool)
                                n7214 = local read "VISA Refnum in\nfor Pump"() -> (w7648:refnum<visa-resource-name>)
                                n7215 = case shown="True" w7647 {
                                frame False {
                                }
                                frame True {
                                n7216 = local read "VISA Refnum in\nfor Pump"() -> (w7649:refnum<visa-resource-name>)
                                n7217 = call "HardStopCurrentProcess (SubVI).vi"("VISA Refnum in"=w7649) -> ()  [unwired: 11 in]
                                }
                                }
                                n7218 = call "ProcessCompletionWaiterWithOutPut (SubVI).vi"("VISA Refnum in"=w7648) -> ("Boolean"=w7646:bool)  [unwired: 10 in]
                                }
                                }
                                frame #5 {
                                n7219 = local read "Buffer-A1 Dispense\nFlow Rate (ul/min) \nfor Equilibration\nof Column-1"() -> (w7653:dbl)
                                n7220 = local read "Buffer-A1 Pumping\nResolution \nfor Equilibration \nof Column-1"() -> (w7652:T2)
                                n7221 = local read "VISA Refnum in\nfor Pump"() -> (w7655:refnum<visa-resource-name>)
                                n7222 = local write "Pause Data Collection"(FALSE ("Pause Data Collection")) -> ()
                                n7223 = local read "Volume of Syringe"() -> (w7654:dbl)
                                n7224 = call "GoToAbsolutePosition(SubVI).vi"("Absolute Volume Position in Syringe (in ul)"=0.0, "Volume of Syringe"=w7654, "Resolution of Pumping"=w7652, "Flow Rate (ul/min)"=w7653, "VISA Refnum in"=w7655) -> ()  [unwired: 6 in, 1 out]
                                }
                                frame #6 {
                                n7225 = local read "Buffer-A1 Pumping\nResolution \nfor Equilibration \nof Column-1"() -> (w7657:T2)
                                n7226 = local read "VISA Refnum in\nfor Pump"() -> (w7659:refnum<visa-resource-name>)
                                n7227 = local read "Initial Plunger Position"() -> (w7658:dbl)
                                n7228 = local read "Volume of Syringe"() -> (w7656:dbl)
                                n7229 = while {
                                tunnel: w7658 -> [w7666]
                                tunnel: w7659 -> [w7665]
                                tunnel: w7657 -> [w7664]
                                tunnel: w7656 -> [w7663]
                                stop <- w7661 stop-if-true
                                n7230 = stacked-sequence {
                                tunnel: w7666 -> [w7673 _]
                                tunnel: w7665 -> [w7672 w7693]
                                tunnel: w7664 -> [w7671 _]
                                tunnel: w7663 -> [w7670 _]
                                tunnel: [_ w7691] -> w7661
                                frame #0 {
                                n7231 = call "AbsolutePlungerPosition (SubVI).vi"("VISA Refnum in"=w7672) -> ("Plunger Position"=w7669:i32)  [unwired: 10 in]
                                n7232 = case shown="\"Standard Pumping\", Default" w7671 {
                                tunnel: w7673 -> [w7678 w7687]
                                tunnel: w7669 -> [w7679 w7686]
                                tunnel: [w7677 w7684] -> w7668
                                tunnel: w7670 -> [w7676 w7685]
                                frame "Standard Pumping", Default {
                                n7233 = Subtract(x=w7678, y=w7679) -> (x-y=w7675:dbl)
                                n7234 = Absolute Value(x=w7675) -> (abs(x)=w7674:dbl)
                                n7235 = Multiply(x=w7674, y=w7676) -> (x*y=w7681:dbl)
                                n7236 = Divide(x=w7681, y=3000.0) -> (x/y=w7677:dbl)
                                }
                                frame "High Resolution Pumping" {
                                n7237 = Subtract(x=w7687, y=w7686) -> (x-y=w7683:dbl)
                                n7238 = Absolute Value(x=w7683) -> (abs(x)=w7682:dbl)
                                n7239 = Multiply(x=w7682, y=w7685) -> (x*y=w7689:dbl)
                                n7240 = Divide(x=w7689, y=24000.0) -> (x/y=w7684:dbl)
                                }
                                }
                                n7241 = local write "Volume being Injected \nin this process"(w7668) -> ()
                                }
                                frame #1 {
                                n7242 = call "LSPOneStatus (SubVI).vi"("VISA Refnum in"=w7693) -> ("read buffer"=w7695:string)  [unwired: 10 in]
                                n7243 = call <vilib>:"Trim Whitespace.vi"("string"=w7695) -> ("trimmed string"=w7694:string)  [unwired: 1 in]
                                n7244 = local read "Stopper that ends \nthe main loops"() -> (w7690:bool)
                                n7245 = Equal?(x=w7694, y="/0`\u0003") -> (x = y?=w7692:bool)
                                n7246 = Or(x=w7692, y=w7690) -> (x .or. y?=w7691:bool)
                                }
                                }
                                n7247 = Wait (ms)(milliseconds to wait=u32 100) -> ()  [unwired: 1 out]
                                n7248 = local read "Stopper that ends \nthe main loops"() -> (w7660:bool)
                                n7249 = case shown="True" w7660 {
                                frame False {
                                }
                                frame True {
                                n7250 = local read "VISA Refnum in\nfor Pump"() -> (w7667:refnum<visa-resource-name>)
                                n7251 = call "HardStopCurrentProcess (SubVI).vi"("VISA Refnum in"=w7667) -> ()  [unwired: 11 in]
                                }
                                }
                                }
                                }
                                frame #7 {
                                # "Change the pump port back to Buffer-A1"
                                n7252 = local read "VISA Refnum in\nfor Pump"() -> (w7698:refnum<visa-resource-name>)
                                n7253 = local read "Port for \nA1-Equilibriation"() -> (w7697:string)
                                n7254 = local write "Pause Data Collection"(TRUE ("Pause Data Collection")) -> ()
                                n7255 = Wait (ms)(milliseconds to wait=u32 500) -> ()  [unwired: 1 out]
                                n7256 = call "PortChanger (SubVI).vi"("Port Number"=w7697, "VISA Refnum in"=w7698) -> ()  [unwired: 10 in]
                                }
                                frame #8 {
                                n7257 = local read "VISA Refnum in\nfor Pump"() -> (w7701:refnum<visa-resource-name>)
                                n7258 = local write "Volume being Injected \nin this process"(0.0 ("Volume being Injected \nin this process")) -> ()
                                n7259 = call "ProcessCompletionWaiter (SubVI).vi"("VISA Refnum in"=w7701) -> ()  [unwired: 11 in]
                                }
                              }
                            }
                            n7260 = local write "Reminder of the \nVolume to be \nPumped"(w7630) -> ()
                          }
                          frame #12 {
                            n7261 = stacked-sequence {
                              frame #0 {
                                n7262 = local read "Buffer-A1 PickUp \nFlow Rate (ul/min)\nfor Equilibration \nof Column-1"() -> (w7705:dbl)
                                n7263 = local read "Buffer-A1 Pumping\nResolution \nfor Equilibration \nof Column-1"() -> (w7704:T2)
                                n7264 = local read "VISA Refnum in\nfor Pump"() -> (w7707:refnum<visa-resource-name>)
                                n7265 = local read "Reminder of the \nVolume to be \nPumped"() -> (w7703:dbl)
                                n7266 = local read "Volume of Syringe"() -> (w7706:dbl)
                                n7267 = call "RPickUp(SubVI).vi"("Volume to be picked up"=w7703, "Volume of Syringe"=w7706, "Resolution of PickUP"=w7704, "PickUp Flow Rate (ul/min)"=w7705, "VISA Refnum in"=w7707) -> ()  [unwired: 6 in, 1 out]
                              }
                              frame #1 {
                                n7268 = while {
                                stop <- w7708 stop-if-true
                                n7269 = local read "Stopper that ends \nthe main loops"() -> (w7709:bool)
                                n7270 = local read "VISA Refnum in\nfor Pump"() -> (w7710:refnum<visa-resource-name>)
                                n7271 = case shown="True" w7709 {
                                frame False {
                                }
                                frame True {
                                n7272 = local read "VISA Refnum in\nfor Pump"() -> (w7711:refnum<visa-resource-name>)
                                n7273 = call "HardStopCurrentProcess (SubVI).vi"("VISA Refnum in"=w7711) -> ()  [unwired: 11 in]
                                }
                                }
                                n7274 = call "ProcessCompletionWaiterWithOutPut (SubVI).vi"("VISA Refnum in"=w7710) -> ("Boolean"=w7708:bool)  [unwired: 10 in]
                                }
                              }
                              frame #2 {
                                # "Reads the initial Plunger Position for computing the volume dispensed"
                                n7275 = local read "VISA Refnum in\nfor Pump"() -> (w7713:refnum<visa-resource-name>)
                                n7276 = call "AbsolutePlungerPosition (SubVI).vi"("VISA Refnum in"=w7713) -> ("Plunger Position"=w7712:i32)  [unwired: 10 in]
                                n7277 = local write "Initial Plunger Position"(w7712) -> ()
                              }
                              frame #3 {
                                # "Switch to Port-2"
                                # "Port-2 of the pump is conncted to column-1 of chip"
                                n7278 = local read "VISA Refnum in\nfor Pump"() -> (w7715:refnum<visa-resource-name>)
                                n7279 = call "PortChanger (SubVI).vi"("Port Number"="2", "VISA Refnum in"=w7715) -> ()  [unwired: 10 in]
                              }
                              frame #4 {
                                n7280 = while {
                                stop <- w7716 stop-if-true
                                n7281 = local read "Stopper that ends \nthe main loops"() -> (w7717:bool)
                                n7282 = local read "VISA Refnum in\nfor Pump"() -> (w7718:refnum<visa-resource-name>)
                                n7283 = case shown="True" w7717 {
                                frame False {
                                }
                                frame True {
                                n7284 = local read "VISA Refnum in\nfor Pump"() -> (w7719:refnum<visa-resource-name>)
                                n7285 = call "HardStopCurrentProcess (SubVI).vi"("VISA Refnum in"=w7719) -> ()  [unwired: 11 in]
                                }
                                }
                                n7286 = call "ProcessCompletionWaiterWithOutPut (SubVI).vi"("VISA Refnum in"=w7718) -> ("Boolean"=w7716:bool)  [unwired: 10 in]
                                }
                              }
                              frame #5 {
                                n7287 = local read "Buffer-A1 Pumping\nResolution \nfor Equilibration \nof Column-1"() -> (w7722:T2)
                                n7288 = local read "Buffer-A1 Dispense\nFlow Rate (ul/min) \nfor Equilibration\nof Column-1"() -> (w7723:dbl)
                                n7289 = local read "VISA Refnum in\nfor Pump"() -> (w7725:refnum<visa-resource-name>)
                                n7290 = local write "Pause Data Collection"(FALSE ("Pause Data Collection")) -> ()
                                n7291 = local read "Volume of Syringe"() -> (w7724:dbl)
                                n7292 = call "GoToAbsolutePosition(SubVI).vi"("Absolute Volume Position in Syringe (in ul)"=0.0 ("Volume to be Dispensed"), "Volume of Syringe"=w7724, "Resolution of Pumping"=w7722, "Flow Rate (ul/min)"=w7723, "VISA Refnum in"=w7725) -> ()  [unwired: 6 in, 1 out]
                              }
                              frame #6 {
                                n7293 = local read "Buffer-A1 Pumping\nResolution \nfor Equilibration \nof Column-1"() -> (w7727:T2)
                                n7294 = local read "VISA Refnum in\nfor Pump"() -> (w7729:refnum<visa-resource-name>)
                                n7295 = local read "Initial Plunger Position"() -> (w7728:dbl)
                                n7296 = local read "Volume of Syringe"() -> (w7726:dbl)
                                n7297 = while {
                                tunnel: w7728 -> [w7736]
                                tunnel: w7729 -> [w7735]
                                tunnel: w7727 -> [w7734]
                                tunnel: w7726 -> [w7733]
                                stop <- w7731 stop-if-true
                                n7298 = stacked-sequence {
                                tunnel: w7736 -> [w7743 _]
                                tunnel: w7735 -> [w7742 w7763]
                                tunnel: w7734 -> [w7741 _]
                                tunnel: w7733 -> [w7740 _]
                                tunnel: [_ w7761] -> w7731
                                frame #0 {
                                n7299 = call "AbsolutePlungerPosition (SubVI).vi"("VISA Refnum in"=w7742) -> ("Plunger Position"=w7739:i32)  [unwired: 10 in]
                                n7300 = case shown="\"Standard Pumping\", Default" w7741 {
                                tunnel: w7743 -> [w7748 w7757]
                                tunnel: w7739 -> [w7749 w7756]
                                tunnel: [w7747 w7754] -> w7738
                                tunnel: w7740 -> [w7746 w7755]
                                frame "Standard Pumping", Default {
                                n7301 = Subtract(x=w7748, y=w7749) -> (x-y=w7745:dbl)
                                n7302 = Absolute Value(x=w7745) -> (abs(x)=w7744:dbl)
                                n7303 = Multiply(x=w7744, y=w7746) -> (x*y=w7751:dbl)
                                n7304 = Divide(x=w7751, y=3000.0) -> (x/y=w7747:dbl)
                                }
                                frame "High Resolution Pumping" {
                                n7305 = Subtract(x=w7757, y=w7756) -> (x-y=w7753:dbl)
                                n7306 = Absolute Value(x=w7753) -> (abs(x)=w7752:dbl)
                                n7307 = Multiply(x=w7752, y=w7755) -> (x*y=w7759:dbl)
                                n7308 = Divide(x=w7759, y=24000.0) -> (x/y=w7754:dbl)
                                }
                                }
                                n7309 = local write "Volume being Injected \nin this process"(w7738) -> ()
                                }
                                frame #1 {
                                n7310 = call "LSPOneStatus (SubVI).vi"("VISA Refnum in"=w7763) -> ("read buffer"=w7765:string)  [unwired: 10 in]
                                n7311 = call <vilib>:"Trim Whitespace.vi"("string"=w7765) -> ("trimmed string"=w7764:string)  [unwired: 1 in]
                                n7312 = local read "Stopper that ends \nthe main loops"() -> (w7760:bool)
                                n7313 = Equal?(x=w7764, y="/0`\u0003") -> (x = y?=w7762:bool)
                                n7314 = Or(x=w7762, y=w7760) -> (x .or. y?=w7761:bool)
                                }
                                }
                                n7315 = Wait (ms)(milliseconds to wait=u32 100) -> ()  [unwired: 1 out]
                                n7316 = local read "Stopper that ends \nthe main loops"() -> (w7730:bool)
                                n7317 = case shown="True" w7730 {
                                frame False {
                                }
                                frame True {
                                n7318 = local read "VISA Refnum in\nfor Pump"() -> (w7737:refnum<visa-resource-name>)
                                n7319 = call "HardStopCurrentProcess (SubVI).vi"("VISA Refnum in"=w7737) -> ()  [unwired: 11 in]
                                }
                                }
                                }
                              }
                              frame #7 {
                                # "Change the pump port to Buffer-C1 for equilibriation of column-2"
                                n7320 = local read "VISA Refnum in\nfor Pump"() -> (w7768:refnum<visa-resource-name>)
                                n7321 = local read "Port for \nC1-Equilibriation"() -> (w7767:string)
                                n7322 = local write "Pause Data Collection"(TRUE ("Pause Data Collection")) -> ()
                                n7323 = Wait (ms)(milliseconds to wait=u32 500) -> ()  [unwired: 1 out]
                                n7324 = call "PortChanger (SubVI).vi"("Port Number"=w7767, "VISA Refnum in"=w7768) -> ()  [unwired: 10 in]
                              }
                              frame #8 {
                                n7325 = local read "VISA Refnum in\nfor Pump"() -> (w7772:refnum<visa-resource-name>)
                                n7326 = local write "Volume being Injected \nin this process"(0.0 ("Volume being Injected \nin this process")) -> ()
